vi "LoadGeneralConfigData.vi"(11 "Refnum in":T1) -> (3 "Refnum out":T1)   [LabVIEW 2014]
uses:
  <vilib>/Utility/config.llb/Config Data RefNum.ctl
  <vilib>/Utility/config.llb/Read Key (I32).vi
  Variables/References.vi
  <vilib>/Utility/config.llb/Write Key (I32).vi
  <vilib>/Utility/config.llb/Read Key (Double).vi
  Variables/Physical data.vi
  <vilib>/Utility/config.llb/Write Key (Double).vi
  <vilib>/Utility/config.llb/NI_LVConfig.lvlib
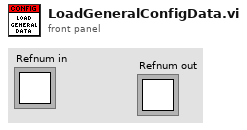
[diagram p1: front panel]
types:
  T1 = typedef "NI_LVConfig.lvlib/Config Data RefNum.ctl" = refnum<k1>
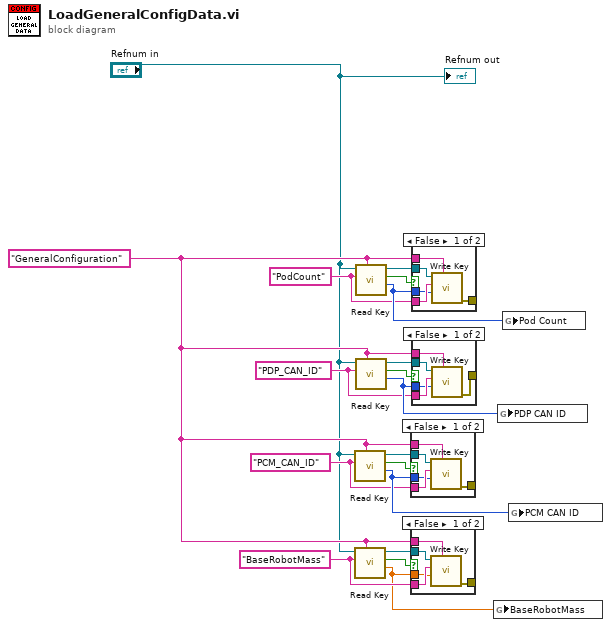
[diagram p0: block diagram]
diagram:
  w6 = "BaseRobotMass" ("string")
  w3 = "GeneralConfiguration" ("name or relative path")
  w10 = "PCM_CAN_ID" ("string")
  w7 = "PDP_CAN_ID" ("string")
  w15 = "PodCount" ("string")
  n1 = call-poly <vilib>:"Read Key.vi"("section"=w3, "key"=w10, "refnum"="Refnum in") -> ("value"=w18:i32, "found?"=w12:bool, "refnum out"=w11:T1)  [unwired: 5 in, 1 out]
  n2 = call-poly <vilib>:"Read Key.vi"("section"=w3, "key"=w6, "refnum"="Refnum in") -> ("value"=w2:dbl, "found?"=w4:bool, "refnum out"=w5:T1)  [unwired: 5 in, 1 out]
  n3 = call-poly <vilib>:"Read Key.vi"("section"=w3, "key"=w15, "refnum"="Refnum in") -> ("value"=w16:i32, "found?"=w13:bool, "refnum out"=w14:T1)  [unwired: 5 in, 1 out]
  n4 = call-poly <vilib>:"Read Key.vi"("section"=w3, "key"=w7, "refnum"="Refnum in") -> ("value"=w17:i32, "found?"=w9:bool, "refnum out"=w8:T1)  [unwired: 5 in, 1 out]
  n5 = case shown="False" w12 {
    tunnel: w11 -> [w23 _]
    tunnel: w10 -> [w22 _]
    tunnel: w18 -> [w21 _]
    tunnel: w3 -> [w20 _]
    tunnel: [w19 _] -> _
    frame False {
      n6 = call-poly <vilib>:"Write Key.vi"("section"=w20, "value"=w21, "key"=w22, "refnum"=w23) -> ("error out"=w19:errorcluster)  [unwired: 5 in, 2 out]
    }
    frame True {
    }
  }
  n7 = case shown="False" w4 {
    tunnel: w5 -> [w28 _]
    tunnel: w6 -> [w27 _]
    tunnel: w2 -> [w26 _]
    tunnel: w3 -> [w25 _]
    tunnel: [w24 _] -> _
    frame False {
      n8 = call-poly <vilib>:"Write Key.vi"("section"=w25, "value"=w26, "key"=w27, "refnum"=w28) -> ("error out"=w24:errorcluster)  [unwired: 5 in, 2 out]
    }
    frame True {
    }
  }
  n9 = case shown="False" w13 {
    tunnel: w14 -> [w33 _]
    tunnel: w15 -> [w32 _]
    tunnel: w16 -> [w31 _]
    tunnel: w3 -> [w30 _]
    tunnel: [w29 _] -> _
    frame False {
      n10 = call-poly <vilib>:"Write Key.vi"("section"=w30, "value"=w31, "key"=w32, "refnum"=w33) -> ("error out"=w29:errorcluster)  [unwired: 5 in, 2 out]
    }
    frame True {
    }
  }
  n11 = case shown="False" w9 {
    tunnel: w8 -> [w38 _]
    tunnel: w7 -> [w37 _]
    tunnel: w17 -> [w36 _]
    tunnel: w3 -> [w35 _]
    tunnel: [w34 _] -> _
    frame False {
      n12 = call-poly <vilib>:"Write Key.vi"("section"=w35, "value"=w36, "key"=w37, "refnum"=w38) -> ("error out"=w34:errorcluster)  [unwired: 5 in, 2 out]
    }
    frame True {
    }
  }
  n13 = global write "Physical data.vi" "BaseRobotMass"(w2) -> ()
  n14 = global write "References.vi" "PDP CAN ID"(w17) -> ()
  n15 = global write "References.vi" "Pod Count"(w16) -> ()
  n16 = global write "References.vi" "PCM CAN ID"(w18) -> ()
  "Refnum out" <- "Refnum in"
